vi "Fluke 289 Read Primary Measurement.vi"() -> ()   [LabVIEW 2015]
doc: "This example shows how to use read a measurement in the Volt/Amp/Hertz mode from the instrument."
uses:
  <instrlib>/Fluke 289/Fluke 289.lvlib
panel:
  out "Attribute":string
  out "State":string
  out "Unit":string
  out "Reading Value":dbl
  in  "VISA resource name":refnum<visa-resource-name>
  # "(c) 2014 National Instruments.  ALL RIGHTS RESERVED."
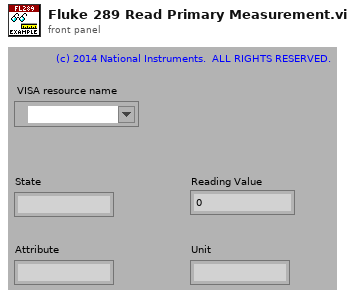
[diagram p1: front panel]
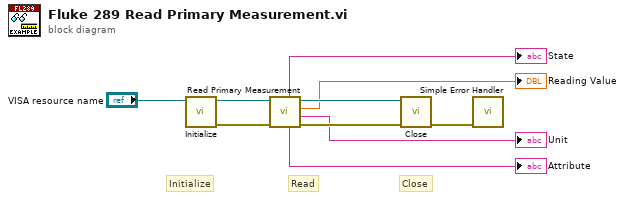
[diagram p0: block diagram]
diagram:
  # "Read"
  # "Close"
  # "Initialize"
  n1 = call <instrlib>:"Initialize.vi"("VISA resource name"="VISA resource name") -> ("error out"=w8:errorcluster, "VISA resource name out"=w9:refnum<visa-resource-name>)  [unwired: 9 in]
  n2 = call <instrlib>:"Read Primary Measurement.vi"("error in (no error)"=w8, "VISA resource name"=w9) -> ("error out"=w6:errorcluster, "Unit"=→"Unit":string, "Reading Value"=→"Reading Value":dbl, "VISA resource name out"=w7:refnum<visa-resource-name>, "Attribute"=→"Attribute":string, "State"=→"State":string)  [unwired: 4 in]
  n3 = call <instrlib>:"Close.vi"("error in (no error)"=w6, "VISA resource name"=w7) -> ("error out"=w5:errorcluster)  [unwired: 9 in]
  n4 = call <vilib>:"Simple Error Handler.vi"("error in (no error)"=w5) -> ()  [unwired: 4 in, 5 out]
